vi "fpga_128ch-SchedulerOV.vi"() -> (0 "overflow":bool, 1 "FIFO Schedule":u8, 2 "Main clock":u32)   [LabVIEW 2011]
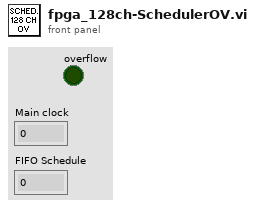
[diagram p1: front panel]
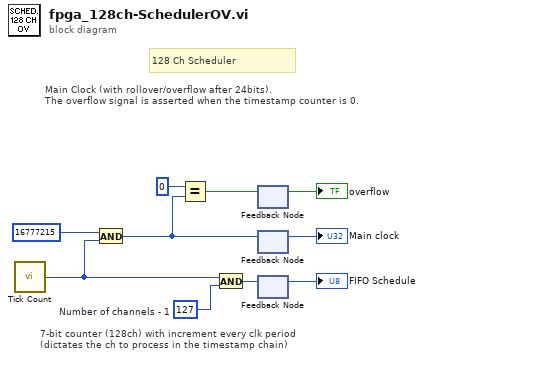
[diagram p0: block diagram]
diagram:
  w10 = u32 127  # Number of channels - 1
  # "128 Ch Scheduler"
  # "Main Clock (with rollover/overflow after 24bits).\nThe overflow signal is asserted when the timestamp counter is 0."
  # "7-bit counter (128ch) with increment every clk period\n(dictates the ch to process in the timestamp chain)"
  n1 = call "Tick Count"() -> ("Tick Count(Ticks)"=w6:u32)
  n2 = And(x=u32 16777215, y=w6) -> (x .and. y?=w5:u32)
  n3 = Equal?(x=u32 0, y=w5) -> (x = y?=w3:bool)
  n4 = And(x=w6, y=w10) -> (x .and. y?=w9:u32)
  n5 = feedback #1() -> (→"overflow":bool)  [unwired: 1 in]
  n6 = feedback-in #1(w3) -> ()
  n7 = feedback-in #2(w5) -> ()
  n8 = feedback #2() -> (→"Main clock":u32)  [unwired: 1 in]
  n9 = feedback-in #3(w9) -> ()
  n10 = feedback #3() -> (→"FIFO Schedule":u32)  [unwired: 1 in]
